vi "Frequency Change Channel 1.vi"(0 "object in":refnum<class "AFG3022B.lvclass">, 3 "Frequency (1000 Hz)":dbl=1000.0, 5 "error in (no error)":errorcluster) -> (14 "object out":refnum<class "AFG3022B.lvclass">, 19 "error out":errorcluster)   [LabVIEW 2023, in "AFG3022B.lvclass"]
uses:
  AFG3022B.lvclass
  AFG3022B.lvclass/AFG3022B.ctl
  <instrlib>/Tektronix AFG 3000 Series/Tektronix AFG 3000 Series.lvlib
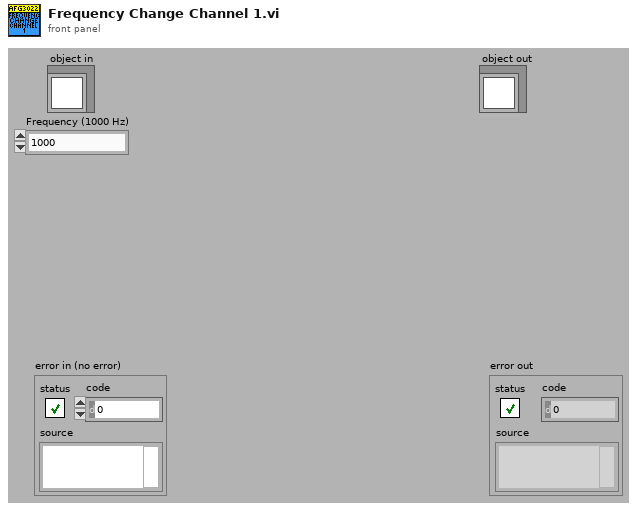
[diagram p1: front panel]
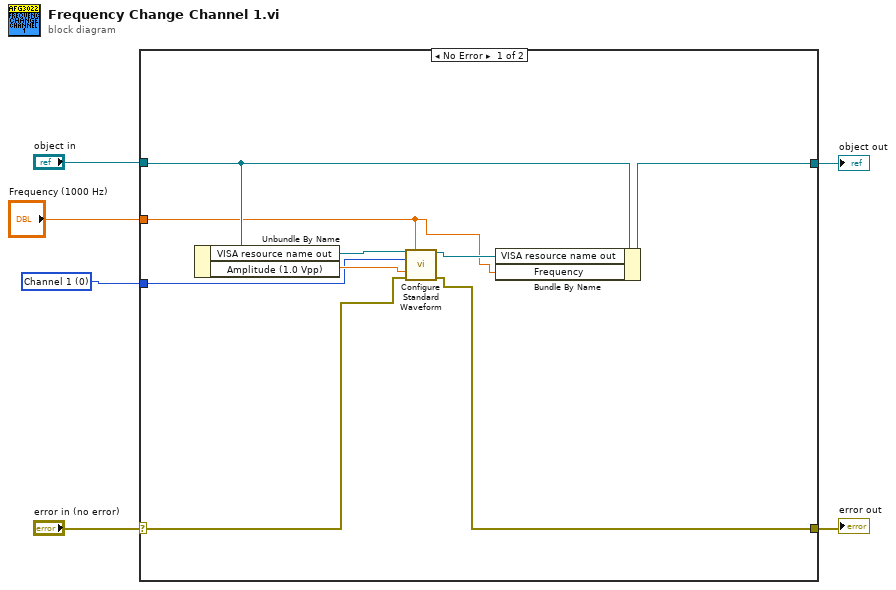
[diagram p0: block diagram]
diagram:
  w1 = u16 0 items=["Channel 1", "Channel 2"] ("Channel (0: Channel 1)")
  n1 = case shown="No Error" "error in (no error)" {
    selector: "error in (no error)" -> [w11 w17]
    tunnel: [w12 w17] -> w5
    tunnel: [w14 w16] -> w3
    tunnel: "object in" -> [w15 w16]
    tunnel: "Frequency (1000 Hz)" -> [w7 _]
    tunnel: w1 -> [w8 _]
    frame No Error {
      n2 = Unbundle By Name(w15) -> ("VISA resource name out"=w9:refnum<visa-resource-name>, "Amplitude (1.0 Vpp)"=w10:dbl)
      n3 = call <instrlib>:"Configure Standard Waveform.vi"("VISA resource name"=w9, "Frequency (1000 Hz)"=w7, "Channel (0: Channel 1)"=w8, "Amplitude (1 Vpp)"=w10, "error in (no error)"=w11) -> ("VISA resource name out"=w13:refnum<visa-resource-name>, "error out"=w12:errorcluster)  [unwired: 9 in]
      n4 = Bundle By Name(cluster=w15, "VISA resource name out"=w13, "Frequency"=w7) -> (w14:refnum<class "AFG3022B.lvclass">)
    }
    frame Error {
    }
  }
  "error out" <- w5
  "object out" <- w3
